vi "ListTidepoolDirectory.vi"(8 "error in (no error)":errorcluster, 10 "Starting Path":string="/pub/outgoing/iridium/", 11 "FTP Server":string="tidepool.nos.noaa.gov") -> (0 "error out":errorcluster, 3 "dir list":T1[](array[typedef]))   [LabVIEW 2014]
uses:
  <vilib>/FTP/ftp2.llb/FTP File Info.ctl
  <vilib>/FTP/NI_FTP.lvlib
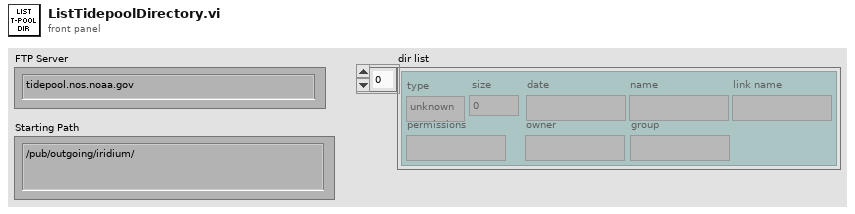
[diagram p1: front panel]
types:
  T1 = typedef "NI_FTP.lvlib/FTP File Info.ctl" = cluster{"type":enum16{"unknown", "file", "dir", "link"}, "permissions":string, "owner":string, "group":string, "size":i32, "date":string, "name":string, "link name":string}
  T2 = typedef "NI_FTP.lvlib/FTP Session.ctl" = refnum<k5>
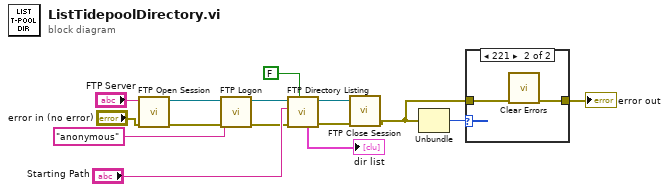
[diagram p0: block diagram]
diagram:
  n1 = call <vilib>:"FTP Open Session.vi"("error in (no error)"="error in (no error)", "address"="FTP Server") -> ("error out"=w5:errorcluster, "ftp session"=w6:T2)  [unwired: 6 in, 2 out]
  n2 = call <vilib>:"FTP Logon.vi"("error in (no error)"=w5, "user"="anonymous", "ftp session"=w6) -> ("error out"=w10:errorcluster, "ftp session out"=w9:T2)  [unwired: 5 in, 2 out]
  n3 = call <vilib>:"FTP Directory Listing.vi"("active (T)"=FALSE, "error in (no error)"=w10, "directory path"="Starting Path", "ftp session"=w9) -> ("error out"=w12:errorcluster, "ftp session out"=w11:T2, "dir list"=→"dir list":T1[])  [unwired: 3 in, 2 out]
  n4 = call <vilib>:"FTP Close Session.vi"("error in (no error)"=w12, "ftp session"=w11) -> ("error out"=w2:errorcluster)  [unwired: 6 in, 3 out]
  n5 = Unbundle(w2) -> ("code"=w3:i32)  [unwired: 2 out]
  n6 = case shown="221" w3 {
    tunnel: w2 -> [w16 w18]
    tunnel: [w16 w17] -> w1
    frame 0, Default {
    }
    frame 221 {
      n7 = call <vilib>:"Clear Errors.vi"("error in (no error)"=w18) -> ("error out"=w17:errorcluster)  [unwired: 5 in, 1 out]
    }
  }
  "error out" <- w1
